vi "获取根目录下所有保存数据文件路径.vi"() -> (1 "文档日期":string[](array[string]), 2 "所有存档数据表路径":path[](array[path]))   [LabVIEW 2014]
uses:
  Global.vi
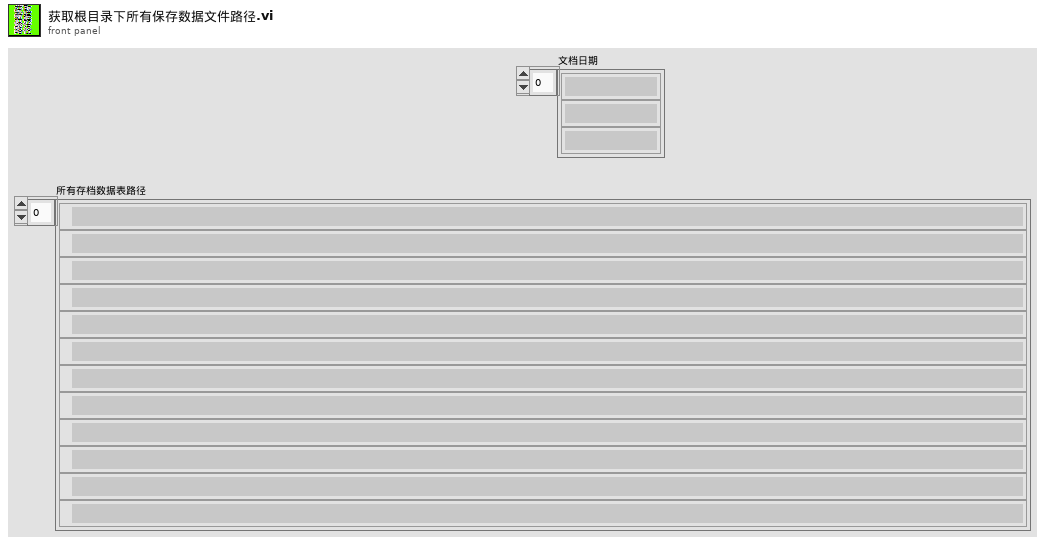
[diagram p1: front panel]
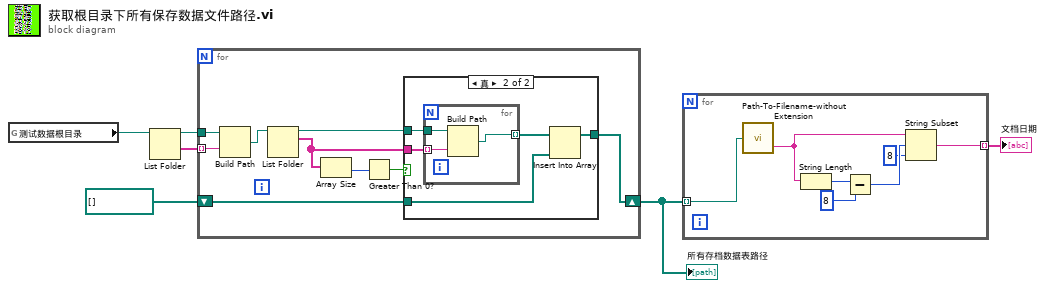
[diagram p0: block diagram]
diagram:
  n1 = global read "Global.vi" "测试数据根目录"() -> (w3:path)
  n2 = List Folder ("罗列文件夹")(path=w3) -> (path out=w5:path, folder names=w4:string[])  [unwired: 3 in, 2 out]
  n3 = for {
    tunnel: w4 -> [w14] mode=indexing
    tunnel: w5 -> [w15]
    shift-right: [w11] -> w2
    shift-left: path[] [] -> [w10]
    n4 = Build Path(base path=w15, name or relative path=w14) -> (appended path=w13:path)
    n5 = List Folder ("罗列文件夹")(path=w13) -> (path out=w12:path, filenames=w9:string[])  [unwired: 3 in, 2 out]
    n6 = Array Size(array=w9) -> (size(s)=w7:i32)
    n7 = Greater Than 0?(x=w7) -> (x > 0?=w8:bool)
    n8 = case shown="真" w8 {
      tunnel: w12 -> [_ w21]
      tunnel: w9 -> [_ w20]
      tunnel: [w16 w18] -> w11
      tunnel: w10 -> [w16 w17]
      frame False {
      }
      frame True {
        n9 = for {
          tunnel: w21 -> [w24]
          tunnel: w20 -> [w23] mode=indexing
          tunnel: [w22] -> w19 mode=indexing
          n10 = Build Path(base path=w24, name or relative path=w23) -> (appended path=w22:path)
        }
        n11 = Insert Into Array(array=w19, new element=w17) -> (w18:path[])  [unwired: 1 in]
      }
    }
  }
  "所有存档数据表路径" <- w2
  n12 = for {
    tunnel: w2 -> [w31] mode=indexing
    tunnel: [w25] -> w1 mode=indexing
    n13 = call "Path-To-Filename-withoutExtension.vi"("Path"=w31) -> ("filename without extension"=w30:string)  [unwired: 1 out]
    n14 = String Length(string=w30) -> (length=w29:i32)
    n15 = Subtract(x=w29, y=8) -> (x-y=w27:i32)
    n16 = String Subset(string=w30, offset (0)=w27, length (rest)=8 ("长度（剩余）")) -> (substring=w25:string)
  }
  "文档日期" <- w1
